vi "ROS_Master_Example.vi"() -> ()   [LabVIEW 2015]
doc: "Starts a ROS master on a given machine"
uses:
  ROS/Code/ROS_Master/ROS_Master.ctl
  ROS/Code/ROS_Master/ROS_Topic.ctl
  ROS/Code/ROS_Master/ROS_Node.ctl
  ROS/Code/ROS_Master/ROS_Service.ctl
  ROS/Code/_ROSDefinition.vi
panel:
  in  "stop":bool
  out "requests":string[](array[string])
  out "TCP received":string
  out "Current":T1
  in  "close":bool
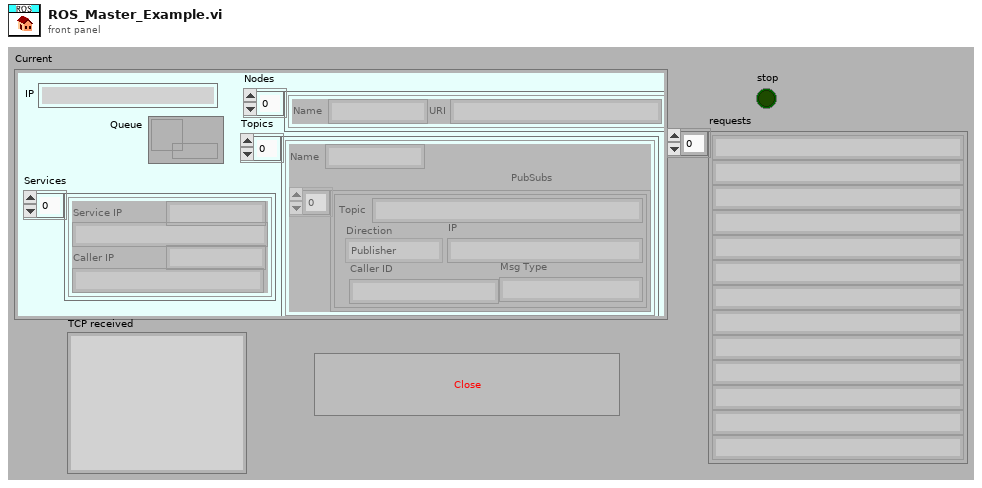
[diagram p1: front panel]
types:
  T1 = typedef "ROS_Master.ctl" = cluster{"IP":string, "Topics":cluster{"Name":string, "PubSubs":T2[]}[], "Nodes":T3[], "Services":T4[], "Queue":refnum<queue>}
  T2 = typedef "ROS_Topic.ctl" = cluster{"Caller ID":string, "IP":string, "Msg Type":string, "Direction":enum16{"Publisher", "Subscriber"}, "Topic":string}
  T3 = typedef "ROS_Node.ctl" = cluster{"Name":string, "URI":string}
  T4 = typedef "ROS_Service.ctl" = cluster{"Service":string, "Service IP":string, "Caller IP":string, "Caller ID":string}
  T5 = cluster{"caller_id":string, "topic":string, "ip":string}
  T6 = cluster{"value":string, "value":string, "value":string}
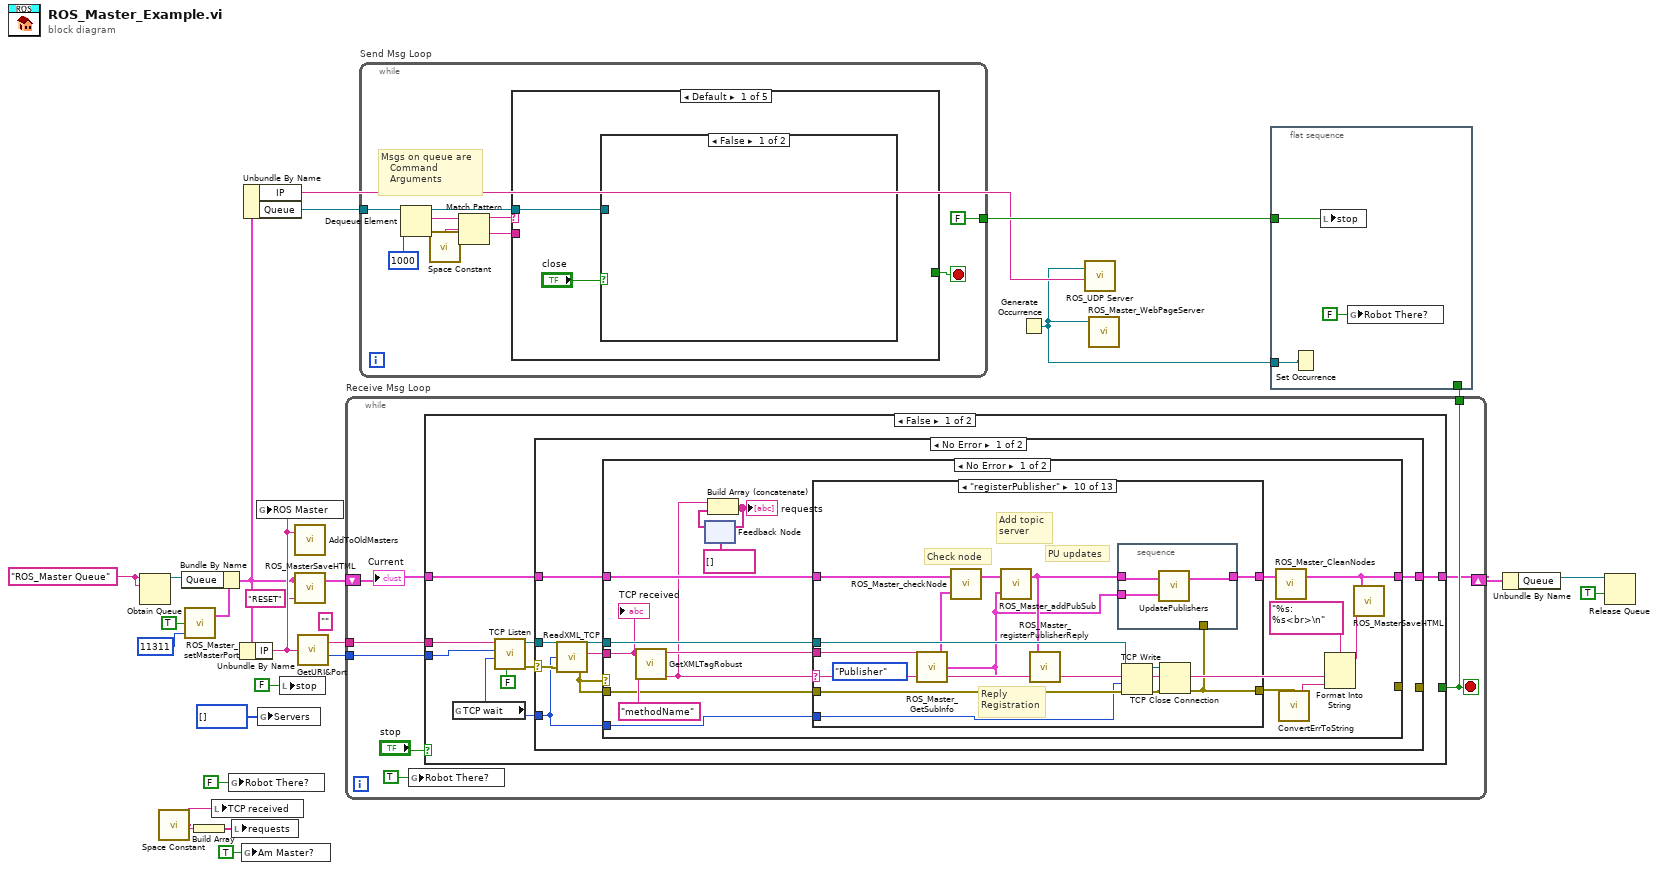
[diagram p0: block diagram]
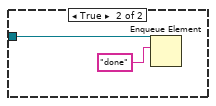
[diagram p2: hidden frame]
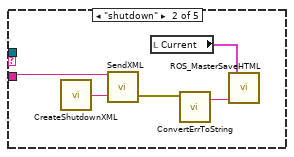
[diagram p3: hidden frame]
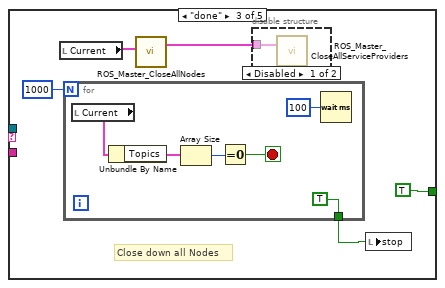
[diagram p4: hidden frame]
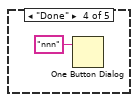
[diagram p6: hidden frame]
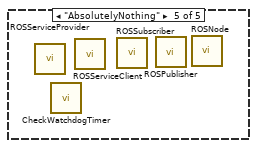
[diagram p7: hidden frame]
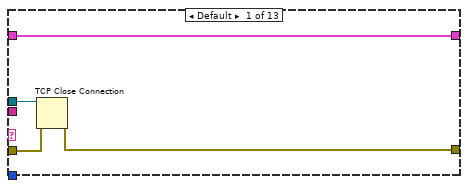
[diagram p8: hidden frame]
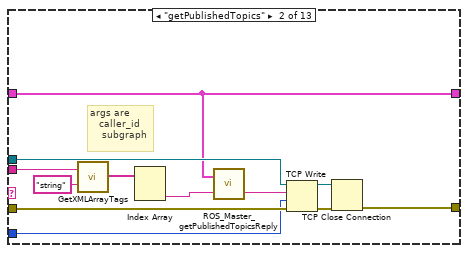
[diagram p9: hidden frame]
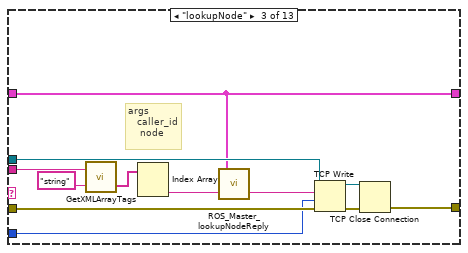
[diagram p10: hidden frame]
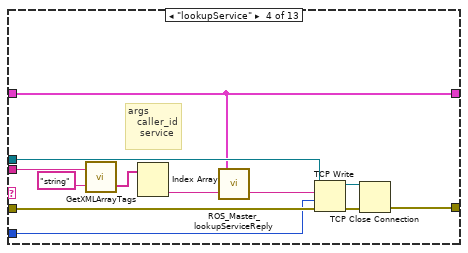
[diagram p11: hidden frame]
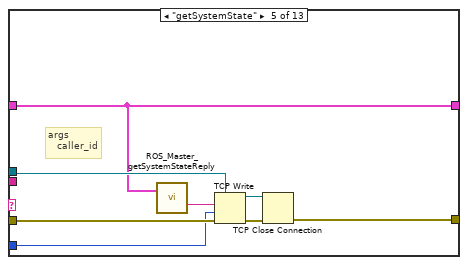
[diagram p12: hidden frame]
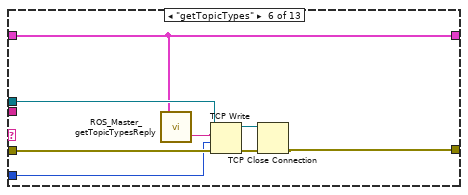
[diagram p13: hidden frame]
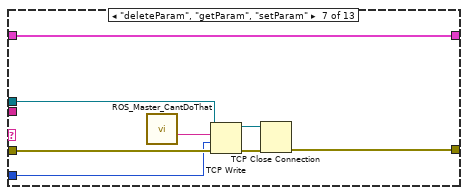
[diagram p14: hidden frame]
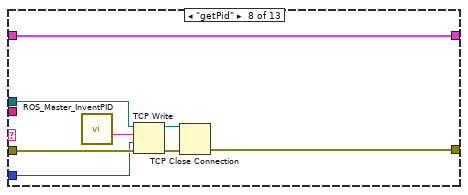
[diagram p15: hidden frame]
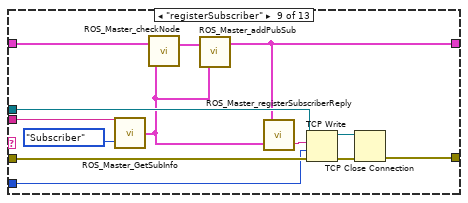
[diagram p16: hidden frame]
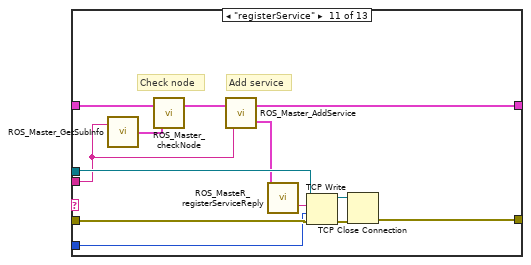
[diagram p17: hidden frame]
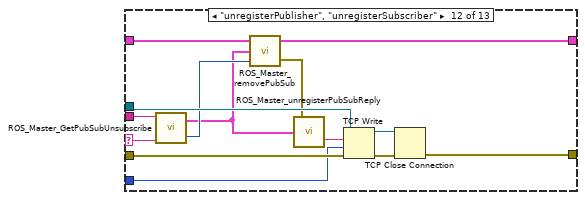
[diagram p18: hidden frame]
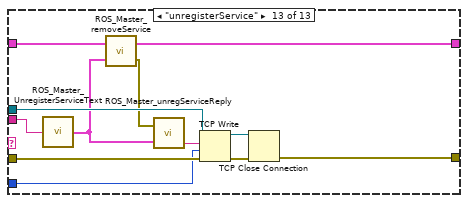
[diagram p19: hidden frame]
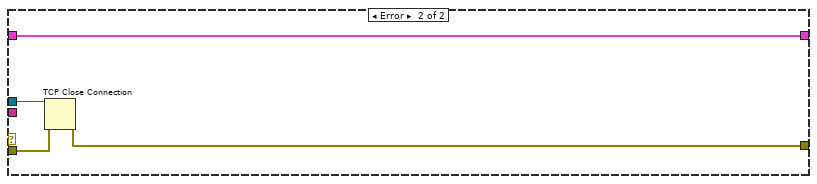
[diagram p20: hidden frame]
diagram:
  (unwired) ""
  w20 = "ROS_Master Queue" ("name (unnamed)")
  n1 = Obtain Queue(name (unnamed)=w20, element data type=w20) -> (queue out=w21:refnum<queue>)  [unwired: 3 in, 2 out]
  n2 = call "Space Constant.vi"() -> ("String"=w18:string)
  n3 = call "ROS_Master_setMasterPort.vi"("Port"=u32 11311, "Wait for real address?"=TRUE) -> ("ROS_Master out"=w19:T1)  [unwired: 2 in]
  n4 = Bundle By Name(cluster=w19, "Queue"=w21) -> (w7:T1)
  n5 = Build Array(w18) -> (w17:string[])
  n6 = local write "TCP received"(w18) -> ()
  n7 = global write "_ROSDefinition.vi" "Robot There?"(FALSE ("Robot There?")) -> ()
  n8 = local write "requests"(w17) -> ()
  n9 = Unbundle By Name(w7) -> ("IP"=w12:string)
  n10 = global write "_ROSDefinition.vi" "Am Master?"(TRUE ("Am Master?")) -> ()
  n11 = Unbundle By Name(w7) -> ("IP"=w8:string, "Queue"=w22:refnum<queue>)
  n12 = global write "_ROSDefinition.vi" "ROS Master"(w12) -> ()
  n13 = global write "_ROSDefinition.vi" "Servers"(u16[] [] ("Servers")) -> ()
  n14 = local write "stop"(FALSE ("stop")) -> ()
  n15 = call "AddToOldMasters.vi"("Address"=w12) -> ()  [unwired: 3 in]
  n16 = call "ROS_MasterSaveHTML.vi"("Latest Request"="RESET", "Current"=w7) -> ()  [unwired: 4 in]
  n17 = call "GetURI&Port.vi"("URI in"=w12) -> ("Port"=w23:u16, "URI"=w24:string)
  n18 = while "Receive Msg Loop" {
    shift-right: [w25] -> w4
    shift-left: w7 -> [w29]
    tunnel: w24 -> [w31]
    tunnel: w23 -> [w30]
    tunnel: [w26] -> w10
    stop <- w26 stop-if-true
    n19 = global write "_ROSDefinition.vi" "Robot There?"(TRUE ("Robot There?")) -> ()
    n20 = case shown="False" "stop" {
      tunnel: w31 -> [w38 _]
      tunnel: w30 -> [w37 _]
      tunnel: [w35 w215] -> w25
      tunnel: w29 -> [w34 w216]
      tunnel: [_ TRUE] -> w26
      frame False {
        n21 = global read "_ROSDefinition.vi" "TCP wait"() -> (w33:i32)
        n22 = call "TCP Listen.vi"("resolve remote address (T)"=FALSE, "timeout ms (wait forever: -1)"=w33, "port"=w37, "service name"=w38) -> ("error out"=w39:errorcluster, "connection ID"=w36:refnum<k5>)  [unwired: 3 in, 3 out]
        n23 = case shown="No Error" w39 {
          selector: w39 -> [w46 w211]
          tunnel: w36 -> [w47 w212]
          tunnel: w34 -> [w44 w213]
          tunnel: [w42 w213] -> w35
          tunnel: w33 -> [w40 _]
          tunnel: [_ w210] -> _
          frame No Error {
            n24 = call "ReadXML_TCP.vi"("error in"=w46, "timeout ms (3000)"=w40, "connection ID in"=w47) -> ("error out"=w41:errorcluster, "data out"=w45:string, "connection ID out"=w43:refnum<k5>)
            n25 = case shown="No Error" w41 {
              tunnel: w45 -> [w49 _]
              tunnel: w44 -> [w62 w209]
              tunnel: w43 -> [w61 w208]
              tunnel: w41 -> [w60 w207]
              tunnel: [w50 w209] -> w42
              tunnel: w40 -> [w56 _]
              tunnel: [_ w206] -> _
              frame No Error {
                n26 = call "GetXMLTagRobust.vi"("Tag"="methodName", "String"=w49) -> ("value"=w48:string, "String w/o Tag"=w63:string)  [unwired: 1 in, 2 out]
                n27 = feedback #1(string[] []) -> (w59:string[])
                n28 = Build Array (concatenate)(w48, w59) -> (w58:string[])
                "requests" <- w58
                n29 = feedback-in #1(w58) -> ()
                n30 = case shown="\"registerPublisher\"" w48 {
                  selector: w48 -> [_ _ _ _ _ _ _ _ _ _ _ w184 _]
                  tunnel: w63 -> [_ w80 w92 w104 _ _ _ _ w149 w159 w167 w185 w205]
                  tunnel: w62 -> [w68 w74 w85 w97 w110 w118 w128 w136 w146 w162 w170 w186 w201]
                  tunnel: [w68 w74 w85 w97 w110 w118 w128 w136 w142 w153 w179 w188 w198] -> w52
                  tunnel: w61 -> [w67 w76 w89 w101 w112 w120 w127 w134 w148 w163 w178 w192 w204]
                  tunnel: w60 -> [w66 w75 w88 w100 w111 w119 w126 w133 w147 w157 w177 w193 w203]
                  tunnel: [w65 w70 w82 w94 w106 w114 w122 w130 w138 w151 w172 w181 w195] -> w55
                  tunnel: w56 -> [_ w69 w81 w93 w105 w113 w121 w129 w137 w150 w171 w180 w194]
                  frame Default {
                    n31 = TCP Close Connection(connection ID=w67, error in (no error)=w66) -> (error out=w65:errorcluster)  [unwired: 1 in, 1 out]
                  }
                  frame "getPublishedTopics" {
                    # "args are\n   caller_id\n    subgraph"
                    n32 = call "GetXMLArrayTags.vi"("ArrayTag"="string", "String"=w80) -> ("Array"=w78:string[])  [unwired: 1 out]
                    n33 = Index Array(array=w78) -> (element #2=w77:string)  [unwired: 2 in, 1 out]
                    n34 = call "ROS_Master_getPublishedTopicsReply.vi"("Subgraph"=w77, "ROS_Master"=w74) -> ("XML"=w73:string)  [unwired: 1 in]
                    n35 = TCP Write(connection ID=w76, data in=w73, error in (no error)=w75, 9:w69) -> (connection ID out=w71:refnum<k5>, error out=w72:errorcluster)  [unwired: 1 out]
                    n36 = TCP Close Connection(connection ID=w71, error in (no error)=w72) -> (error out=w70:errorcluster)  [unwired: 1 in, 1 out]
                  }
                  frame "lookupNode" {
                    # "args\n   caller_id\n    node"
                    n37 = call "GetXMLArrayTags.vi"("ArrayTag"="string", "String"=w92) -> ("Array"=w90:string[])  [unwired: 1 out]
                    n38 = Index Array(array=w90) -> (element #2=w87:string)  [unwired: 2 in, 1 out]
                    n39 = call "ROS_Master_lookupNodeReply.vi"("node"=w87, "ROS_Master in"=w85) -> ("XML"=w86:string)  [unwired: 1 in]
                    n40 = TCP Write(connection ID=w89, data in=w86, error in (no error)=w88, 9:w81) -> (connection ID out=w83:refnum<k5>, error out=w84:errorcluster)  [unwired: 1 out]
                    n41 = TCP Close Connection(connection ID=w83, error in (no error)=w84) -> (error out=w82:errorcluster)  [unwired: 1 in, 1 out]
                  }
                  frame "lookupService" {
                    # "args\n   caller_id\n    service"
                    n42 = call "GetXMLArrayTags.vi"("ArrayTag"="string", "String"=w104) -> ("Array"=w102:string[])  [unwired: 1 out]
                    n43 = Index Array(array=w102) -> (element #2=w99:string)  [unwired: 2 in, 1 out]
                    n44 = call "ROS_Master_lookupServiceReply.vi"("Service"=w99, "ROS_Master in"=w97) -> ("XML"=w98:string)  [unwired: 1 in]
                    n45 = TCP Write(connection ID=w101, data in=w98, error in (no error)=w100, 9:w93) -> (connection ID out=w95:refnum<k5>, error out=w96:errorcluster)  [unwired: 1 out]
                    n46 = TCP Close Connection(connection ID=w95, error in (no error)=w96) -> (error out=w94:errorcluster)  [unwired: 1 in, 1 out]
                  }
                  frame "getSystemState" {
                    # "args\n   caller_id"
                    n47 = call "ROS_Master_getSystemStateReply.vi"("ROS_Master in"=w110) -> ("XML"=w109:string)  [unwired: 2 in]
                    n48 = TCP Write(connection ID=w112, data in=w109, error in (no error)=w111, 9:w105) -> (connection ID out=w107:refnum<k5>, error out=w108:errorcluster)  [unwired: 1 out]
                    n49 = TCP Close Connection(connection ID=w107, error in (no error)=w108) -> (error out=w106:errorcluster)  [unwired: 1 in, 1 out]
                  }
                  frame "getTopicTypes" {
                    n50 = call "ROS_Master_getTopicTypesReply.vi"("ROS_Master in"=w118) -> ("Topics XML"=w117:string)  [unwired: 2 in]
                    n51 = TCP Write(connection ID=w120, data in=w117, error in (no error)=w119, 9:w113) -> (connection ID out=w115:refnum<k5>, error out=w116:errorcluster)  [unwired: 1 out]
                    n52 = TCP Close Connection(connection ID=w115, error in (no error)=w116) -> (error out=w114:errorcluster)  [unwired: 1 in, 1 out]
                  }
                  frame "deleteParam", "getParam", "setParam" {
                    n53 = call "ROS_Master_CantDoThat.vi"() -> ("XML"=w125:string)
                    n54 = TCP Write(connection ID=w127, data in=w125, error in (no error)=w126, 9:w121) -> (connection ID out=w123:refnum<k5>, error out=w124:errorcluster)  [unwired: 1 out]
                    n55 = TCP Close Connection(connection ID=w123, error in (no error)=w124) -> (error out=w122:errorcluster)  [unwired: 1 in, 1 out]
                  }
                  frame "getPid" {
                    n56 = call "ROS_Master_InventPID.vi"() -> ("XML"=w135:string)  [unwired: 3 in]
                    n57 = TCP Write(connection ID=w134, data in=w135, error in (no error)=w133, 9:w129) -> (connection ID out=w131:refnum<k5>, error out=w132:errorcluster)  [unwired: 1 out]
                    n58 = TCP Close Connection(connection ID=w131, error in (no error)=w132) -> (error out=w130:errorcluster)  [unwired: 1 in, 1 out]
                  }
                  frame "registerSubscriber" {
                    n59 = call "ROS_Master_GetSubInfo.vi"("Direction"=enum16{"Publisher", "Subscriber"}."Subscriber", "String w/o Tag"=w149) -> ("PubSub"=w144:T2)
                    n60 = call "ROS_Master_checkNode.vi"("PubSub"=w144, "ROS_Master in"=w146) -> ("ROS_Master out"=w145:T1)  [unwired: 1 in]
                    n61 = call "ROS_Master_addPubSub.vi"("PubSub"=w144, "ROS_Master in"=w145) -> ("ROS_Master out"=w142:T1)  [unwired: 1 in]
                    n62 = call "ROS_Master_registerSubscriberReply.vi"("PubSub"=w144, "ROS_Master in"=w142) -> ("XML"=w143:string)  [unwired: 1 in]
                    n63 = TCP Write(connection ID=w148, data in=w143, error in (no error)=w147, 9:w137) -> (connection ID out=w139:refnum<k5>, error out=w140:errorcluster)  [unwired: 1 out]
                    n64 = TCP Close Connection(connection ID=w139, error in (no error)=w140) -> (error out=w138:errorcluster)  [unwired: 1 in, 1 out]
                  }
                  frame "registerPublisher" {
                    # "PU updates"
                    # "Reply\nRegistration"
                    # "Add topic\nserver"
                    # "Check node"
                    n65 = call "ROS_Master_GetSubInfo.vi"("Direction"=enum16{"Publisher", "Subscriber"}."Publisher", "String w/o Tag"=w159) -> ("PubSub"=w152:T2)
                    n66 = call "ROS_Master_checkNode.vi"("PubSub"=w152, "ROS_Master in"=w162) -> ("ROS_Master out"=w161:T1)  [unwired: 1 in]
                    n67 = call "ROS_Master_addPubSub.vi"("PubSub"=w152, "ROS_Master in"=w161) -> ("ROS_Master out"=w154:T1)  [unwired: 1 in]
                    n68 = call "ROS_Master_registerPublisherReply.vi"("PubSub"=w152, "ROS_Master in"=w154) -> ("XML"=w160:string)  [unwired: 1 in]
                    n69 = TCP Write(connection ID=w163, data in=w160, error in (no error)=w157, 9:w150) -> (connection ID out=w156:refnum<k5>, error out=w155:errorcluster)  [unwired: 1 out]
                    n70 = TCP Close Connection(connection ID=w156, error in (no error)=w155) -> (error out=w151:errorcluster)  [unwired: 1 in, 1 out]
                    n71 = stacked-sequence {
                      tunnel: w154 -> [w166]
                      tunnel: [w165] -> w153
                      tunnel: w152 -> [w164]
                      tunnel: w151 -> [_]
                      frame #0 {
                        n72 = call "UpdatePublishers.vi"("PubSub"=w164, "ROS_Master in"=w166) -> ("ROS_Master out"=w165:T1)  [unwired: 1 in]
                      }
                    }
                  }
                  frame "registerService" {
                    # "Add service"
                    # "Check node"
                    n73 = call "ROS_Master_GetSubInfo.vi"("String w/o Tag"=w167) -> ("PubSub"=w168:T2)  [unwired: 1 in]
                    n74 = call "ROS_Master_checkNode.vi"("PubSub"=w168, "ROS_Master in"=w170) -> ("ROS_Master out"=w169:T1)  [unwired: 1 in]
                    n75 = call "ROS_Master_AddService.vi"("String w/o Tag"=w167, "ROS_Master in"=w169) -> ("Service"=w176:T4, "ROS_Master out"=w179:T1)
                    n76 = call "ROS_MasteR_registerServiceReply.vi"("Service"=w176) -> ("XML"=w175:string)  [unwired: 2 in]
                    n77 = TCP Write(connection ID=w178, data in=w175, error in (no error)=w177, 9:w171) -> (connection ID out=w173:refnum<k5>, error out=w174:errorcluster)  [unwired: 1 out]
                    n78 = TCP Close Connection(connection ID=w173, error in (no error)=w174) -> (error out=w172:errorcluster)  [unwired: 1 in, 1 out]
                  }
                  frame "unregisterPublisher", "unregisterSubscriber" {
                    n79 = call "ROS_Master_GetPubSubUnsubscribe.vi"("Value"=w184, "String w/o Tag"=w185) -> ("Direction"=w191:enum16{"Publisher", "Subscriber"}, "PubSub"=w190:T5)
                    n80 = call "ROS_Master_removePubSub.vi"("Direction"=w191, "PubSub"=w190, "ROS_Master in"=w186) -> ("error out"=w189:errorcluster, "ROS_Master our"=w188:T1)
                    n81 = call "ROS_Master_unregisterPubSubReply.vi"("PubSub"=w190, "error in"=w189) -> ("XML"=w187:string)  [unwired: 1 in]
                    n82 = TCP Write(connection ID=w192, data in=w187, error in (no error)=w193, 9:w180) -> (connection ID out=w182:refnum<k5>, error out=w183:errorcluster)  [unwired: 1 out]
                    n83 = TCP Close Connection(connection ID=w182, error in (no error)=w183) -> (error out=w181:errorcluster)  [unwired: 1 in, 1 out]
                  }
                  frame "unregisterService" {
                    n84 = call "ROS_Master_UnregisterServiceText.vi"("String w/o Tag"=w205) -> ("Cluster"=w200:T6)
                    n85 = call "ROS_Master_removeService.vi"("Service"=w200, "ROS_Master in"=w201) -> ("error out"=w199:errorcluster, "ROS_Master out"=w198:T1)
                    n86 = call "ROS_Master_unregServiceReply.vi"("Service"=w200, "error in"=w199) -> ("XML"=w202:string)  [unwired: 1 in]
                    n87 = TCP Write(connection ID=w204, data in=w202, error in (no error)=w203, 9:w194) -> (connection ID out=w196:refnum<k5>, error out=w197:errorcluster)  [unwired: 1 out]
                    n88 = TCP Close Connection(connection ID=w196, error in (no error)=w197) -> (error out=w195:errorcluster)  [unwired: 1 in, 1 out]
                  }
                }
                n89 = call "ROS_Master_CleanNodes.vi"("ROS_Master in"=w52) -> ("ROS_Master out"=w50:T1)  [unwired: 2 in]
                n90 = call "ConvertErrToString.vi"("error in (no error)"=w55) -> ("String"=w54:string)  [unwired: 1 out]
                n91 = Format Into String(format string="%s:  %s<br>\n", w48, w54) -> (resulting string=w51:string)  [unwired: 2 in, 1 out]
                n92 = call "ROS_MasterSaveHTML.vi"("Latest Request"=w51, "Current"=w50) -> ()  [unwired: 4 in]
                "TCP received" <- w49
              }
              frame Error {
                n93 = TCP Close Connection(connection ID=w208, error in (no error)=w207) -> (error out=w206:errorcluster)  [unwired: 1 in, 1 out]
              }
            }
          }
          frame Error {
            n94 = TCP Close Connection(connection ID=w212, error in (no error)=w211) -> (error out=w210:errorcluster)  [unwired: 1 in, 1 out]
          }
        }
      }
      frame True {
        # "Otherwise never updates FP"
        n95 = Bundle By Name(cluster=w216, "Nodes"=T3[] []) -> (w215:T1)
        n96 = local write "Current"(w215) -> ()
        n97 = call "ROS_MasterSaveHTML.vi"("Latest Request"="Master Stopped <br>", "Current"=w215) -> ()  [unwired: 4 in]
      }
    }
    "Current" <- w29
  }
  n98 = while "Send Msg Loop" {
    tunnel: w22 -> [w227]
    tunnel: [FALSE ("stop")] -> w16
    stop <- w221 stop-if-true
    # "Msgs on queue are\n   Command\n   Arguments"
    n99 = Dequeue Element(queue=w227, timeout in ms (-1)=1000) -> (queue out=w219:refnum<queue>, element=w225:string)  [unwired: 1 in, 2 out]
    n100 = call "Space Constant.vi"() -> ("String"=w224:string)
    n101 = Match Pattern(string=w225, regular expression=w224) -> (before substring=w223:string, after substring=w222:string)  [unwired: 1 in, 2 out]
    n102 = case shown="Default" w223 {
      tunnel: w222 -> [_ w236 _ _ _]
      tunnel: [_ _ TRUE _ _] -> w221
      tunnel: w219 -> [w228 _ _ _ _]
      frame Default {
        n103 = case shown="False" "close" {
          tunnel: w228 -> [_ w230]
          frame False {
          }
          frame True {
            n104 = Enqueue Element(queue=w230, element="done") -> ()  [unwired: 2 in, 3 out]
          }
        }
      }
      frame "shutdown" {
        n105 = call "CreateShutdownXML.vi"() -> ("XML"=w235:string)  [unwired: 3 in]
        n106 = call "SendXML.vi"("Send"=w235, "URI in"=w236) -> ("error out"=w234:errorcluster)  [unwired: 1 out]
        n107 = local read "Current"() -> (w233:T1)
        n108 = call "ConvertErrToString.vi"("error in (no error)"=w234) -> ("String"=w232:string)  [unwired: 1 out]
        n109 = call "ROS_MasterSaveHTML.vi"("Latest Request"=w232, "Current"=w233) -> ()  [unwired: 4 in]
      }
      frame "done" {
        # "Close down all Nodes"
        n110 = local read "Current"() -> (w237:T1)
        n111 = for {
          N: 1000 -> [_]
          tunnel: [TRUE ("stop")] -> w238
          stop <- w243 stop-if-true
          n112 = local read "Current"() -> (w246:T1)
          n113 = Unbundle By Name(w246) -> ("Topics"=w245:cluster{"Name":string, "PubSubs":T2[]}[])
          n114 = Array Size(array=w245) -> (size(s)=w244:i32)
          n115 = Equal To 0?(x=w244) -> (x = 0?=w243:bool)
          n116 = Wait (ms)(milliseconds to wait=u32 100) -> ()  [unwired: 1 out]
        }
        n117 = call "ROS_Master_CloseAllNodes.vi"("Current Master"=w237) -> ()  [unwired: 3 in]
        n118 = disable-structure shown="Disabled" {
          disable-tunnel: w237 -> [w241 _]
          frame Disabled {
            n119 = call "ROS_Master_CloseAllServiceProviders.vi"("Current Master"=w241) -> ()  [unwired: 3 in]
          }
          frame Enabled {
          }
        }
        n120 = local write "stop"(w238) -> ()
      }
      frame "Done" {
        n121 = One Button Dialog(message="nnn") -> ()  [unwired: 1 in, 1 out]
      }
      frame "AbsolutelyNothing" {
        n122 = call "ROSServiceProvider.vi"() -> ()  [unwired: 4 in]
        n123 = call "CheckWatchdogTimer.vi"() -> ()  [unwired: 6 in]
        n124 = call "ROSServiceClient.vi"() -> ()  [unwired: 4 in]
        n125 = call "ROSSubscriber.vi"() -> ()  [unwired: 4 in]
        n126 = call "ROSPublisher.vi"() -> ()  [unwired: 4 in]
        n127 = call "ROSNode.vi"() -> ()  [unwired: 4 in]
      }
    }
  }
  n128 = Generate Occurrence() -> (w1:refnum<k4>)
  n129 = call "ROS_UDP Server.vi"("IP"=w8, "Occurrence in"=w1) -> ()  [unwired: 2 in]
  n130 = call "ROS_Master_WebPageServer.vi"("occurrence"=w1) -> ()  [unwired: 5 in]
  n131 = flat-sequence {
    tunnel: w16 -> [w251]
    tunnel: w10 -> [_]
    tunnel: w1 -> [w249]
    frame #0 {
      n132 = Set Occurrence(w249) -> ()
      n133 = local write "stop"(w251) -> ()
      n134 = global write "_ROSDefinition.vi" "Robot There?"(FALSE ("Robot There?")) -> ()
    }
  }
  n135 = Unbundle By Name(w4) -> ("Queue"=w2:refnum<queue>)
  n136 = Release Queue(queue=w2, force destroy? (F)=TRUE) -> ()  [unwired: 1 in, 3 out]
